vi "write metadata.vi"(8 "error in":errorcluster, 10 "metadata":string, 11 "system tag in":refnum<class "tag descriptor.lvclass">) -> (0 "error out":errorcluster, 3 "system tag out":refnum<class "tag descriptor.lvclass">)   [LabVIEW 2013, in "tag bus.lvlib" / "tag descriptor.lvclass"]
doc: "Writes the metadata field in a tag descriptor. This field can be used for any user-defined information, like a description."
uses:
  tag descriptor.lvclass
  tag descriptor.lvclass/tag descriptor.ctl
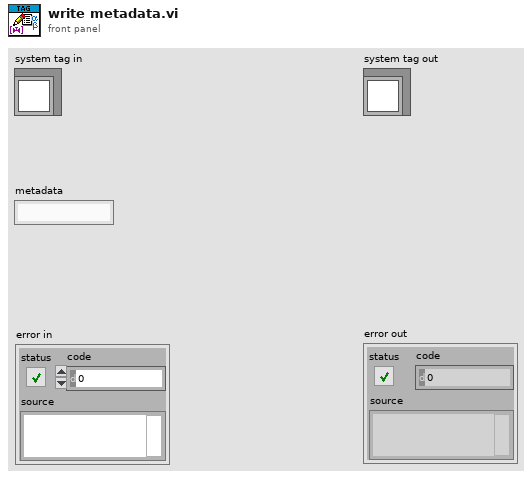
[diagram p1: front panel]
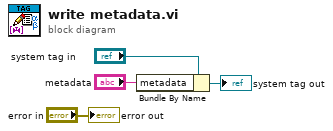
[diagram p0: block diagram]
diagram:
  n1 = Bundle By Name(cluster="system tag in", "metadata"="metadata") -> (→"system tag out":refnum<class "tag descriptor.lvclass">)
  "error out" <- "error in"
